vi "WaitForData.vi"(8 "error in (no error)":errorcluster, 11 "Connection in":refnum<class "Connection.lvclass">) -> (0 "error out":errorcluster, 3 "Connection out":refnum<class "Connection.lvclass">)   [LabVIEW 2022 SP3, in "Connection.lvlib" / "Connection.lvclass"]
uses:
  Connection.lvclass
  C:/Users/jakub/repos/gh/sw4sys/lv-tcp-server-sample/LoggingActor/Source/LoggingActor/LoggingActor/LoggingActor.lvclass
  C:/Program Files (x86)/National Instruments/LabVIEW 2022/vi.lib/ActorFramework/Actor/Actor.lvclass
  Connection.lvclass/Connection.ctl
  LoggingActor/Source/LoggingActor/LoggingActor/LoggingActor.lvclass/LoggingActor.ctl
  <vilib>/ActorFramework/Actor/Actor.lvclass/Actor.ctl
  <vilib>/ActorFramework/Message Enqueuer/Message Enqueuer.lvclass/Message Enqueuer.ctl
  CallerMessage Messages/ConnectionDataRead Msg/ConnectionDataRead Msg.lvclass/ConnectionDataRead Msg.ctl
  LoggingActor/Source/LoggingActor/LoggingActor/Read Logger.vi
  <vilib>/ActorFramework/Message Enqueuer/Init from Existing Queue.vi
  <vilib>/ActorFramework/Message Enqueuer/Enqueue.vi
  CallerMessage Messages/ConnectionDataRead Msg/ConnectionDataRead Msg.lvclass
  C:/Program Files (x86)/National Instruments/LabVIEW 2022/vi.lib/ActorFramework/Message/Message.lvclass
  Connection Messages/WaitForData Msg/WaitForData Msg.lvclass
  Connection Messages/Kill Msg/Kill Msg.lvclass
  <vilib>/ActorFramework/Message Priority Queue/Priority Enqueue.vi
  Logger/Source/Logger/Logger.lvclass
  <vilib>/ActorFramework/Message Enqueuer/Message Enqueuer.lvclass
  TcpSocket/Source/TcpSocket/Connection/Connection.lvclass
  <vilib>/ActorFramework/Actor/Actor.lvclass
  ReadData/ReadData.lvclass
  StringUtils/Source/StringUtils/StringUtils.lvlib
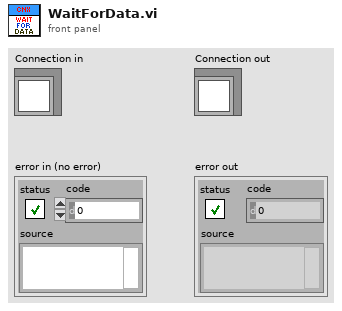
[diagram p1: front panel]
types:
  T1 = typedef "Connection.lvlib/Connection.lvclass/_State.ctl" = enum16{"WaitForInit", "Active", "Dying"}
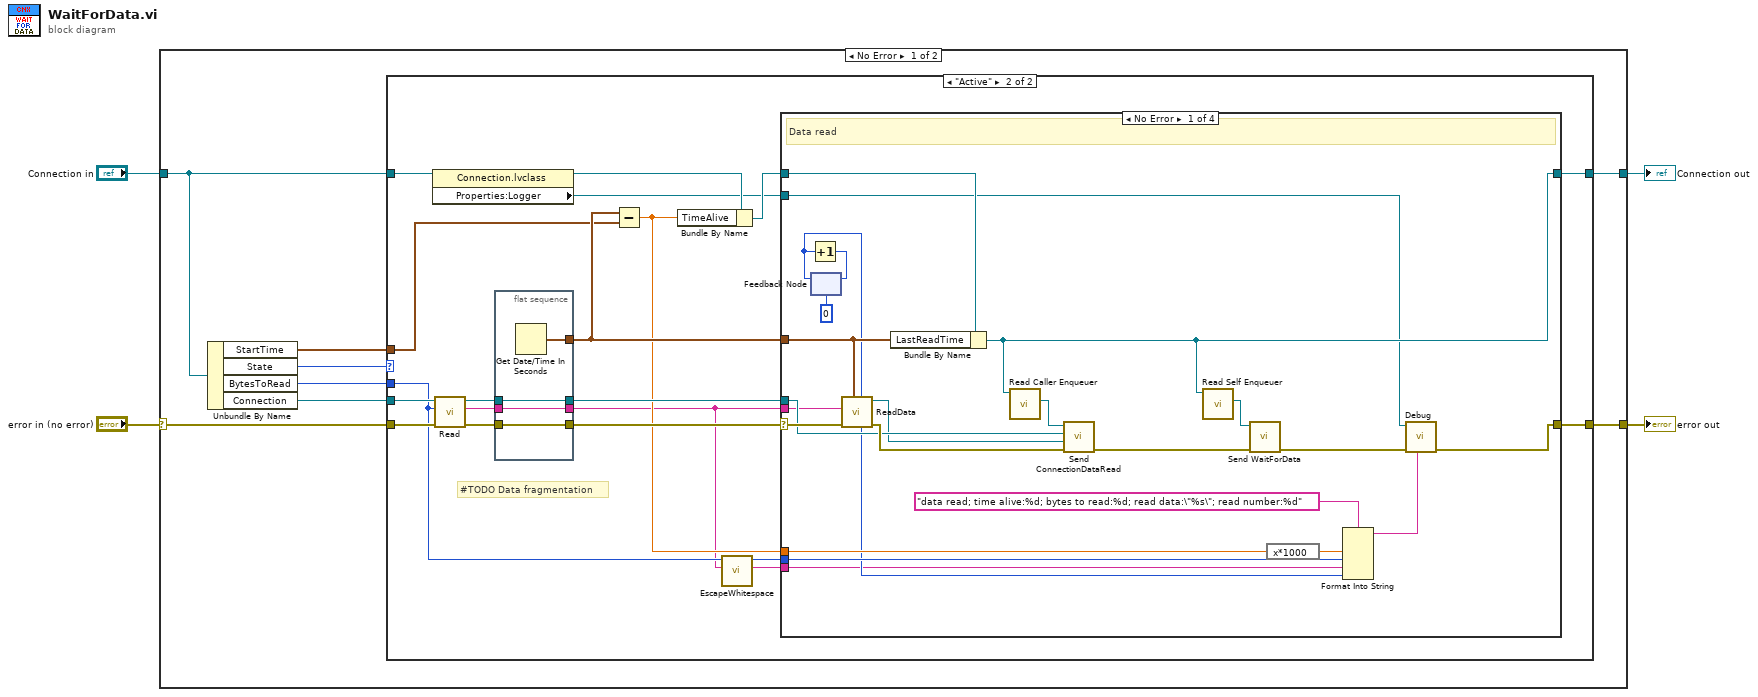
[diagram p0: block diagram]
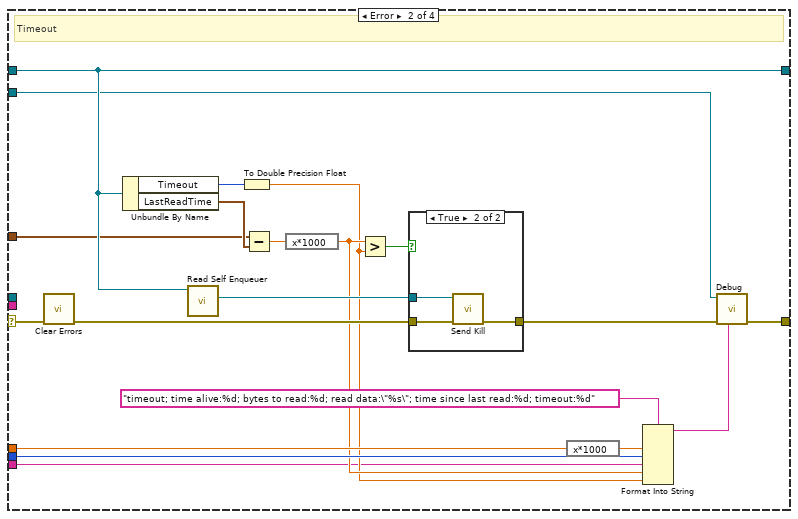
[diagram p3: hidden frame]
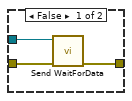
[diagram p4: hidden frame]
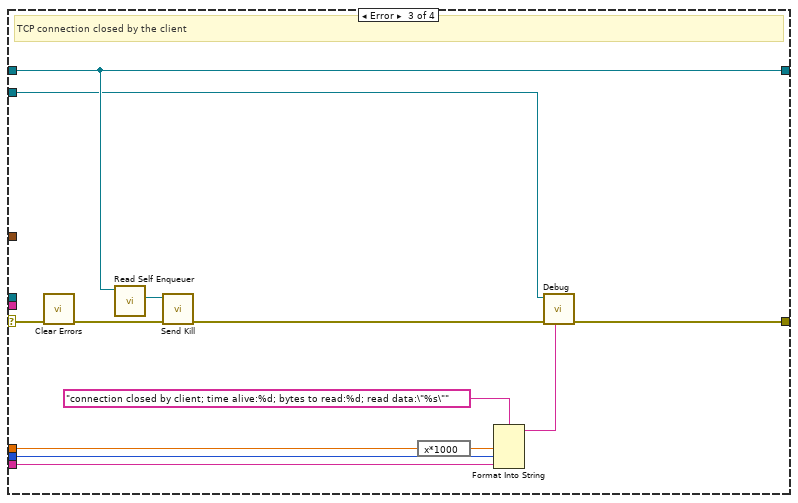
[diagram p5: hidden frame]
diagram:
  n1 = case shown="No Error" "error in (no error)" {
    selector: "error in (no error)" -> [w10 w103]
    tunnel: [w9 w103] -> w3
    tunnel: [w8 w102] -> w1
    tunnel: "Connection in" -> [w5 w102]
    frame No Error {
      n2 = Unbundle By Name(w5) -> ("StartTime"=w7:timestamp, "State"=w6:T1, "BytesToRead"=w11:i32, "Connection"=w12:refnum<class "Connection.lvclass">)
      n3 = case shown="\"Active\"" w6 {
        tunnel: w12 -> [_ w33]
        tunnel: w11 -> [_ w21]
        tunnel: w10 -> [w13 w32]
        tunnel: [w13 w20] -> w9
        tunnel: [w14 w17] -> w8
        tunnel: w7 -> [_ w26]
        tunnel: w5 -> [w14 w25]
        frame Default {
        }
        frame "Active" {
          # "#TODO Data fragmentation"
          n4 = property class="Connection.lvclass"(reference=w25) -> (reference out=w16:refnum<class "Connection.lvclass">, "Properties:Logger"=w15:refnum<class "Logger.lvclass">)  [unwired: 1 in, 1 out]
          n5 = call-dynamic "Read.vi"("error in (no error)"=w32, "BytesToRead"=w21, "Connection in"=w33) -> ("error out"=w30:errorcluster, "Data"=w29:string, "Connection out"=w23:refnum<class "Connection.lvclass">)  [unwired: 6 in]
          n6 = flat-sequence {
            tunnel: [w37] -> w31
            tunnel: w30 -> [w37]
            tunnel: [w36] -> w18
            tunnel: w29 -> [w36]
            tunnel: [w35] -> w28
            tunnel: [w34] -> w24
            tunnel: w23 -> [w34]
            frame #0 {
              n7 = Get Date/Time In Seconds() -> (seconds since 1Jan1904=w35:timestamp)
            }
          }
          n8 = Subtract(x=w28, y=w26) -> (x-y=w22:dbl)
          n9 = Bundle By Name(cluster=w16, "TimeAlive"=w22) -> (w27:refnum<class "Connection.lvclass">)
          n10 = call "EscapeWhitespace.vi"("InputString"=w18) -> ("EscapedWhitespace"=w19:string)  [unwired: 10 in]
          n11 = case shown="No Error" w31 {
            selector: w31 -> [w59 w76 w99 w101]
            tunnel: [w38 w63 w89 w101] -> w20
            tunnel: [w49 w74 w97 w100] -> w17
            tunnel: w27 -> [w60 w74 w97 w100]
            tunnel: w18 -> [w46 _ _ _]
            tunnel: w28 -> [w58 w72 _ _]
            tunnel: w24 -> [w53 _ _ _]
            tunnel: w22 -> [w45 w68 w92 _]
            tunnel: w21 -> [w43 w67 w91 _]
            tunnel: w19 -> [w41 w64 w90 _]
            tunnel: w15 -> [w39 w61 w87 _]
            frame No Error {
              # "Data read"
              n12 = feedback #1(u32 0) -> (w42:u32)
              n13 = Increment(x=w42) -> (x+1=w56:u32)
              n14 = feedback-in #1(w56) -> ()
              n15 = call "ReadData.vi"("ReadNumber"=w42, "TimeStamp"=w58, "error in (no error)"=w59, "Data"=w46) -> ("error out"=w55:errorcluster, "ReadData"=w52:refnum<class "ReadData.lvclass">)  [unwired: 6 in]
              n16 = Bundle By Name(cluster=w60, "LastReadTime"=w58) -> (w49:refnum<class "Connection.lvclass">)
              n17 = call <vilib>:"Read Caller Enqueuer.vi"("Actor"=w49) -> ("Caller Enqueuer"=w54:refnum<class "Message Enqueuer.lvclass">)  [unwired: 10 in]
              n18 = call "Send ConnectionDataRead.vi"("error in (no error)"=w55, "ReadData"=w52, "Connection"=w53, "Message Enqueuer"=w54) -> ("error out"=w51:errorcluster)  [unwired: 6 in, 1 out]
              n19 = call <vilib>:"Read Self Enqueuer.vi"("Actor"=w49) -> ("Self Enqueuer"=w48:refnum<class "Message Enqueuer.lvclass">)  [unwired: 10 in]
              n20 = call "Send WaitForData.vi"("error in (no error)"=w51, "Message Enqueuer"=w48) -> ("error out"=w50:errorcluster)  [unwired: 8 in, 1 out]
              n21 = expression code="x*1000"(w45) -> (w44:dbl)
              n22 = Format Into String(format string="data read; time alive:%d; bytes to read:%d; read data:\"%s\"; read number:%d", w44, w43, w41, w42) -> (resulting string=w40:string)  [unwired: 2 in, 1 out]
              n23 = call-dynamic "Debug.vi"("Message"=w40, "error in (no error)"=w50, "Logger in"=w39) -> ("error out"=w38:errorcluster)  [unwired: 5 in, 1 out]
            }
            frame Error {
              # "Timeout"
              n24 = call <vilib>:"Clear Errors.vi"("error in (no error)"=w76) -> ("error out"=w71:errorcluster)  [unwired: 5 in, 1 out]
              n25 = Unbundle By Name(w74) -> ("Timeout"=w78:i32, "LastReadTime"=w80:timestamp)
              n26 = call <vilib>:"Read Self Enqueuer.vi"("Actor"=w74) -> ("Self Enqueuer"=w73:refnum<class "Message Enqueuer.lvclass">)  [unwired: 10 in]
              n27 = To Double Precision Float(number=w78) -> (double precision float=w65:dbl)
              n28 = Subtract(x=w72, y=w80) -> (x-y=w79:dbl)
              n29 = expression code="x*1000"(w79) -> (w66:dbl)
              n30 = Greater?(x=w66, y=w65) -> (0:w75:bool)
              n31 = case shown="True" w75 {
                tunnel: [w83 w85] -> w77
                tunnel: w71 -> [w82 w84]
                tunnel: w73 -> [w81 w86]
                frame False {
                  n32 = call "Send WaitForData.vi"("error in (no error)"=w82, "Message Enqueuer"=w81) -> ("error out"=w83:errorcluster)  [unwired: 8 in, 1 out]
                }
                frame True {
                  n33 = call "Send Kill.vi"("error in (no error)"=w84, "Message Enqueuer"=w86) -> ("error out"=w85:errorcluster)  [unwired: 8 in, 1 out]
                }
              }
              n34 = expression code="x*1000"(w68) -> (w70:dbl)
              n35 = Format Into String(format string="timeout; time alive:%d; bytes to read:%d; read data:\"%s\"; time since last read:%d; timeout:%d", w70, w67, w64, w66, w65) -> (resulting string=w62:string)  [unwired: 2 in, 1 out]
              n36 = call-dynamic "Debug.vi"("Message"=w62, "error in (no error)"=w77, "Logger in"=w61) -> ("error out"=w63:errorcluster)  [unwired: 5 in, 1 out]
            }
            frame Error {
              # "TCP connection closed by the client"
              n37 = call <vilib>:"Clear Errors.vi"("error in (no error)"=w99) -> ("error out"=w98:errorcluster)  [unwired: 5 in, 1 out]
              n38 = call <vilib>:"Read Self Enqueuer.vi"("Actor"=w97) -> ("Self Enqueuer"=w95:refnum<class "Message Enqueuer.lvclass">)  [unwired: 10 in]
              n39 = call "Send Kill.vi"("error in (no error)"=w98, "Message Enqueuer"=w95) -> ("error out"=w96:errorcluster)  [unwired: 8 in, 1 out]
              n40 = expression code="x*1000"(w92) -> (w94:dbl)
              n41 = Format Into String(format string="connection closed by client; time alive:%d; bytes to read:%d; read data:\"%s\"", w94, w91, w90) -> (resulting string=w88:string)  [unwired: 2 in, 1 out]
              n42 = call-dynamic "Debug.vi"("Message"=w88, "error in (no error)"=w96, "Logger in"=w87) -> ("error out"=w89:errorcluster)  [unwired: 5 in, 1 out]
            }
            frame Default {
              # "Error"
            }
          }
        }
      }
    }
    frame Error {
    }
  }
  "error out" <- w3
  "Connection out" <- w1
